vi "PH_Cam_BaseClass.PC get Frame Rate.vi"(0 "i ref in":refnum<vi>, 2 "on":bool, 5 "error in (no error)":errorcluster) -> (14 "i ref out":refnum<vi>, 19 "error out":errorcluster)   [LabVIEW 2014, in "PH_Cam_BaseClass.lvlib"]
doc: "This VI sets a few Attributes and GUI elements."
uses:
  PH_Cam_BaseClass.lvlib
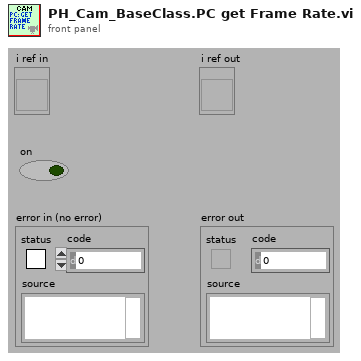
[diagram p1: front panel]
types:
  T1 = typedef "PH_Cam_BaseClass.lvlib/PH_Cam_BaseClass.i attribute.ctl" = cluster{"Gui Refs":T2, "Cam":cluster{"Source Notifier":refnum<notifier>, "Error":errorcluster, "Camera ID":string}, "Images":cluster{"Cam":T3, "Operation":T3, "PSDB":T3}, "Window Image":cluster{"Indicate Image":bool, "Window No.":i32, "Scale Facor":dbl, "Center Cross":bool, "Subtract Backgr":bool, "CoG":bool, "Color Palette":cluster{"Red":u8, "Green":u8, "Blue":u8}[], "Image On":bool}, "Default Prdc Int":i32, "Performance":cluster{"on":bool, "Timestamp Last Frame":i32}, "Histogram":cluster{"on":bool, "Mapping":bool}, "Save Image":cluster{"Save":bool, "File refnum":refnum<file>}, "Setting Service ID":i32, "Screen":cluster{"x-resolution":i16, "y-resolution":i16}, "On":bool, "Constructor finished":bool, "configured":bool}
  T2 = typedef "PH_Cam_BaseClass.lvlib/PH_Cam_BaseClass.GUI Refs.ctl" = cluster{"Frame Rate":refnum<vi>, "Get Frame Rate":refnum<vi>, "Show Image":refnum<vi>, "Get Histogram":refnum<vi>, "Mapping":refnum<vi>, "Histogram":refnum<vi>, "Center Cross":refnum<vi>, "Center of Gravity":refnum<vi>, "Scale Factor [%]":refnum<vi>, "Save Image":refnum<vi>, "Palette":refnum<vi>, "Subtract Background":refnum<vi>, "Cam Error":refnum<vi>, "On":refnum<vi>, "Cam List":refnum<vi>}
  T3 = typedef "IMAQ Image.ctl" = refnum<image>
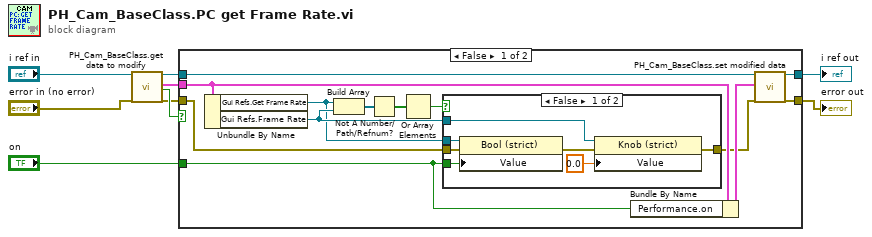
[diagram p0: block diagram]
diagram:
  n1 = call "PH_Cam_BaseClass.get data to modify.vi"("i ref in"="i ref in", "error in (no error)"="error in (no error)") -> ("i ref out"=w5:refnum<vi>, "i attribute"=w7:T1, "timed out"=w9:bool, "error out"=w3:errorcluster)  [unwired: 14 in]
  n2 = case shown="False" w9 {
    tunnel: w3 -> [w17 w31]
    tunnel: [w22 w31] -> w4
    tunnel: w5 -> [w21 w32]
    tunnel: [w20 w32] -> w6
    tunnel: w7 -> [w18 _]
    tunnel: "on" -> [w16 _]
    frame False {
      n3 = Unbundle By Name(w18) -> ("Gui Refs.Get Frame Rate"=w10:refnum<vi>, "Gui Refs.Frame Rate"=w11:refnum<vi>)
      n4 = Build Array(w10, w11) -> (w14:refnum<vi>[])
      n5 = Not A Number/Path/Refnum?(number/path/refnum=w14) -> (NaN/Path/Refnum?=w13:bool[])
      n6 = Or Array Elements(Boolean array=w13) -> (logical OR=w12:bool)
      n7 = case shown="False" w12 {
        tunnel: w17 -> [w29 w30]
        tunnel: [w26 w30] -> w15
        tunnel: w16 -> [w28 _]
        tunnel: w11 -> [w25 _]
        tunnel: w10 -> [w24 _]
        frame False {
          n8 = property class="Bool (strict)"(reference=w24, error in=w29, "Value"=w28) -> (error out=w27:errorcluster)  [unwired: 1 out]
          n9 = property class="Knob (strict)"(reference=w25, error in=w27, "Value"=0.0) -> (error out=w26:errorcluster)  [unwired: 1 out]
        }
        frame True {
        }
      }
      n10 = Bundle By Name(cluster=w18, "Performance.on"=w16) -> (w19:T1)
      n11 = call "PH_Cam_BaseClass.set modified data.vi"("i ref in"=w21, "i attribute"=w19, "error in (no error)"=w15) -> ("i ref out"=w20:refnum<vi>, "error out"=w22:errorcluster)  [unwired: 15 in]
    }
    frame True {
    }
  }
  "i ref out" <- w6
  "error out" <- w4
